vi "verify_results_array.vi"(7 "Mesured values":dbl[](array[numeric]) format="%#_6p", 8 "error in":errorcluster, 9 "Lower Limit":dbl[](array[numeric]), 10 "Upper Limit":dbl[](array[numeric]), 11 "comparison":T2 caption="Enum") -> (0 "error out":errorcluster, 2 "Pass or fail array":bool[](array[boolean]), 3 "Array":T1(array[cluster]))   [LabVIEW 2021]
uses:
  controls/comparison selection.ctl
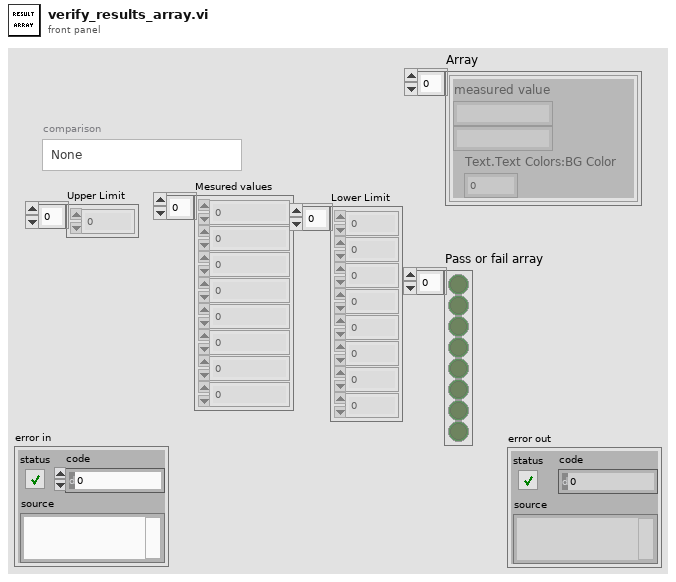
[diagram p1: front panel]
types:
  T1 = cluster{"measured value":string, string, "Text.Text Colors:BG Color":u32}[]
  T2 = typedef "comparison selection.ctl" = enum16{"None", "in-range?", "less than?", "greater than?", "equal to?", "not equal to?", "less or equal to?", "greater or equal to?"}
  T3 = cluster{"measured value":string, string, "Text.Text Colors:BG Color":u32}
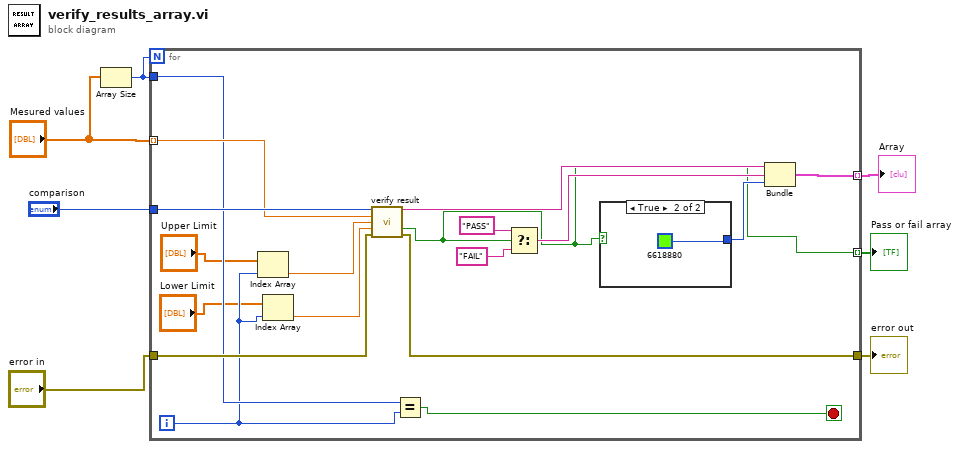
[diagram p0: block diagram]
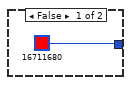
[diagram p2: hidden frame]
diagram:
  n1 = Array Size(array="Mesured values") -> (size(s)=w3:i32)
  n2 = for {
    N: w3 -> [_]
    tunnel: "Mesured values" -> [w20] mode=indexing
    tunnel: [w25] -> w1 mode=indexing
    tunnel: "comparison" -> [w24]
    tunnel: w3 -> [w15]
    tunnel: "error in" -> [w21]
    tunnel: [w22] -> w5
    tunnel: [w9] -> w2 mode=indexing
    i -> [w12]
    stop <- w14 stop-if-true
    n3 = Index Array(array="Upper Limit", index=w12) -> (element=w8:dbl)
    n4 = Index Array(array="Lower Limit", index=w12) -> (element=w10:dbl)
    n5 = call "verify result.vi"("comparison"=w24, "measured data"=w20, "UL"=w8, "LL"=w10, "error in (no error)"=w21) -> ("measured value"=w23:string, "result?"=w9:bool, "error out"=w22:errorcluster)  [unwired: 7 in, 1 out]
    n6 = Equal?(x=w15, y=w12) -> (x = y?=w14:bool)
    n7 = Select(t="PASS", s=w9, f="FAIL") -> (s? t:f=w17:string)
    n8 = case shown="True" w9 {
      tunnel: [u32 16711680 ("Text.Text Colors:BG Color") u32 6618880 ("Text.Text Colors:BG Color")] -> w16
      frame False {
      }
      frame True {
      }
    }
    n9 = Bundle("measured value"=w23, w17, "Text.Text Colors:BG Color"=w16) -> (w25:T3)  [unwired: 1 in]
  }
  "error out" <- w5
  "Pass or fail array" <- w2
  "Array" <- w1
